vi "Dispatch Shutdown.vi"(8 "error in (no error)":errorcluster, 11 "Dispatcher in":refnum<class "Dispatcher Thread.lvclass">) -> (0 "error out":errorcluster, 3 "Dispatcher out":refnum<class "Dispatcher Thread.lvclass">)   [LabVIEW 2017, in "DSF Core.lvlib" / "Dispatcher Thread.lvclass"]
uses:
  Dispatcher Thread.lvclass
  C:/Git/DSF/Data Sharing Framework/Source/Core/Engine/Classes/Thread/Thread.lvclass
  Thread/Thread.lvclass
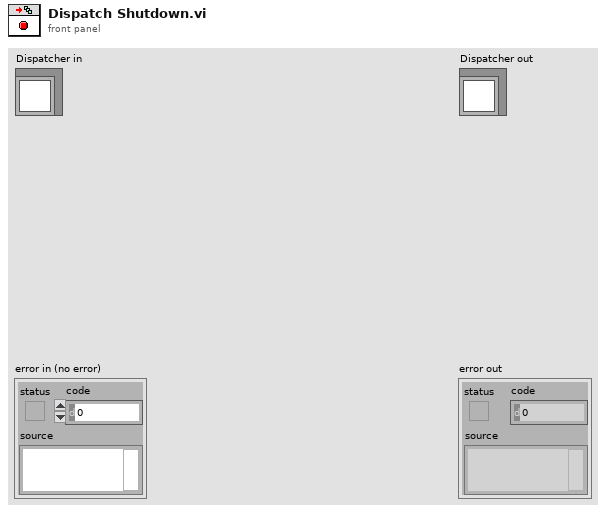
[diagram p1: front panel]
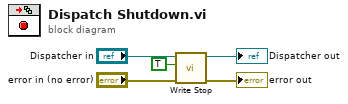
[diagram p0: block diagram]
diagram:
  n1 = call "Write Stop.vi"("error in (no error)"="error in (no error)", "stop"=TRUE, "Thread in"="Dispatcher in") -> ("error out"=→"error out":errorcluster, "Thread out"=→"Dispatcher out":refnum<class "Dispatcher Thread.lvclass">)  [unwired: 7 in]
